vi "runPushing.vi"(4 "Service? in":bool, 5 "Distance":dbl, 6 "Fault?":bool, 7 "Time":dbl, 8 "error in (no error)":errorcluster, 9 "Actuators in":T1, 10 "State in":T2, 11 "SystemsCheck in":refnum<class "SystemsCheck.lvclass">) -> (0 "error out":errorcluster, 1 "Actuators out":T1, 2 "State out":T2, 3 "SystemsCheck out":refnum<class "SystemsCheck.lvclass">)   [LabVIEW 2017, in "ControlLibrary.lvlib" / "SystemsCheck.lvclass"]
uses:
  SystemsCheck.lvclass
  TypeDef_ControlState.ctl
  TypeDef_DigitalOuts.ctl
  RunTypeClass/RunType.lvclass
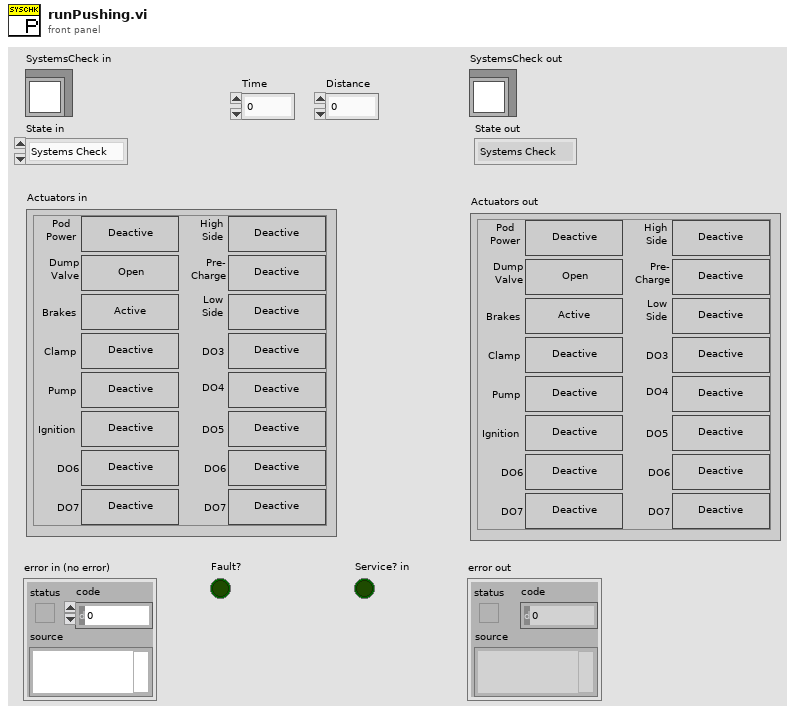
[diagram p1: front panel]
types:
  T1 = typedef "TypeDef_DigitalOuts.ctl" = cluster{"Pod Power":bool, "Dump Valve":bool, "Brakes":bool, "Clamp":bool, "Pump":bool, "Ignition":bool, "DO6":bool, "DO7":bool, "HighSide":bool, "Precharge":bool, "LowSide":bool, "DO3":bool, "DO4":bool, "DO5":bool, "DO62":bool, "DO72":bool}
  T2 = typedef "TypeDef_ControlState.ctl" = enum16{"Systems Check", "Idle", "Ready", "Pushing", "Coast", "Braking", "Fault", "Shutdown", "Service", "Precharge", "Blank"}
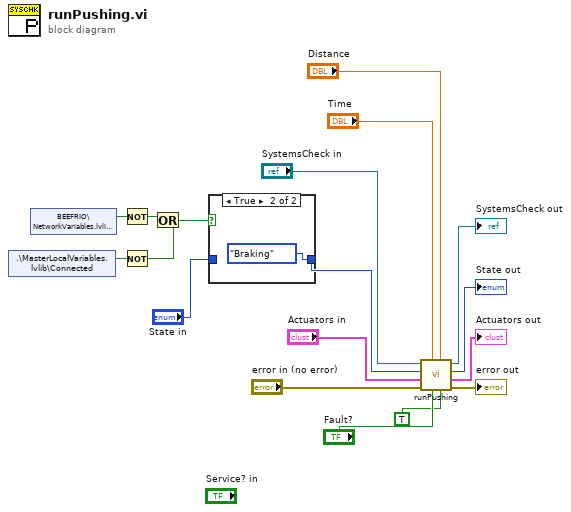
[diagram p0: block diagram]
diagram:
  n1 = shared-variable ".\\MasterLocalVariables.lvlib\\Connected"() -> (w3:bool)  [unwired: 1 in, 1 out]
  n2 = shared-variable "BEEFRIO\\NetworkVariables.lvlib\\Service"() -> (w4:bool)  [unwired: 1 in, 1 out]
  n3 = Not(x=w4) -> (.not. x?=w2:bool)
  n4 = Not(x=w3) -> (.not. x?=w1:bool)
  n5 = Or(x=w2, y=w1) -> (x .or. y?=w5:bool)
  n6 = case shown="True" w5 {
    tunnel: [w19 TypeDef_ControlState."Braking" ("State in")] -> w7
    tunnel: "State in" -> [w19 _]
    frame False {
    }
    frame True {
    }
  }
  n7 = call-parent "runPushing.vi"("Service? in"=TRUE, "Distance"="Distance", "Fault?"="Fault?", "Time"="Time", "error in (no error)"="error in (no error)", "Actuators in"="Actuators in", "State in"=w7, "RunType in"="SystemsCheck in") -> ("error out"=→"error out":errorcluster, "Actuators out"=→"Actuators out":T1, "State out"=→"State out":T2, "RunType out"=→"SystemsCheck out":refnum<class "SystemsCheck.lvclass">)
